vi "CRYPIC Change Sate.vi"(11 "sAction":string) -> (3 "sData_Out":string)   [LabVIEW 2013]
uses:
  CRYMain Sub Window Global.vi
  DataView/VIEW/CRYNew View Global.vi
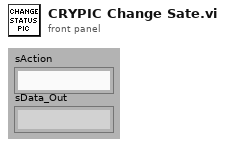
[diagram p1: front panel]
types:
  T1 = enum8{"Enabled", "Disabled", "Disabled and Grayed Out"}
  T2 = typedef "Graph Main Info Cluster.ctl" = cluster{"Selected_BarIdx":i32, "Selected_PanelIdx":i32, "Graph Main VIRef":refnum<vi>, "ToolBarClick":bool, "Spliter Ref Array":refnum<vi>[], "Panel Ref Array":refnum<vi>[], "Spliter_matrix":i32[][], "Panel_matrix":i32[][], "child_spliterIdx_matrix":i32[][], "split_pos_matrix":i32[][], "Title State":bool, "sQueueName":string, "Frame nID":i32, "Graph VIRef Array":cluster{"Graph VIRef":refnum<vi>, "Panel Idx":i32, "Frame VIRef":refnum<vi>, "Icon Ring":i32, "Graph Type":string}[], "View Type":string}
  T3 = typedef "LVRectTypeDef.ctl" = cluster{"Left":i16, "Top":i16, "Right":i16, "Bottom":i16}
  T4 = cluster{"nID":i32[], "Frame":cluster{"nType":i32, "nParent":i32, "pVIW":refnum<vi>, "pSPW":refnum<vi>, "nTypeF":i32, "pVIF":refnum<vi>, "pSPF":refnum<vi>, "nIDSpliter":i32, "nProperty":i32, "Bound":T3, "nID":i32, "nData":i32, "sData":string, "pWVI":refnum<vi>, "sTitle":string, "cPages":cluster{"nPage":i32, "sTitle":string, "sIcon":string, "pVI":refnum<vi>, "nID":i32}[], "pTab":refnum<vi>, "nIDPages":i32[], "pSPT":refnum<vi>, "sTemp":string, "nDockID":i32, "nDockLR":i32, "sIcon":string}[]}
  T5 = cluster{"nType":i32, "nParent":i32, "pVIW":refnum<vi>, "pSPW":refnum<vi>, "nTypeF":i32, "pVIF":refnum<vi>, "pSPF":refnum<vi>, "nIDSpliter":i32, "nProperty":i32, "Bound":T3, "nID":i32, "nData":i32, "sData":string, "pWVI":refnum<vi>, "sTitle":string, "cPages":cluster{"nPage":i32, "sTitle":string, "sIcon":string, "pVI":refnum<vi>, "nID":i32}[], "pTab":refnum<vi>, "nIDPages":i32[], "pSPT":refnum<vi>, "sTemp":string, "nDockID":i32, "nDockLR":i32, "sIcon":string}[]
  T6 = cluster{"Graph VIRef":refnum<vi>, "Panel Idx":i32, "Frame VIRef":refnum<vi>, "Icon Ring":i32, "Graph Type":string}[]
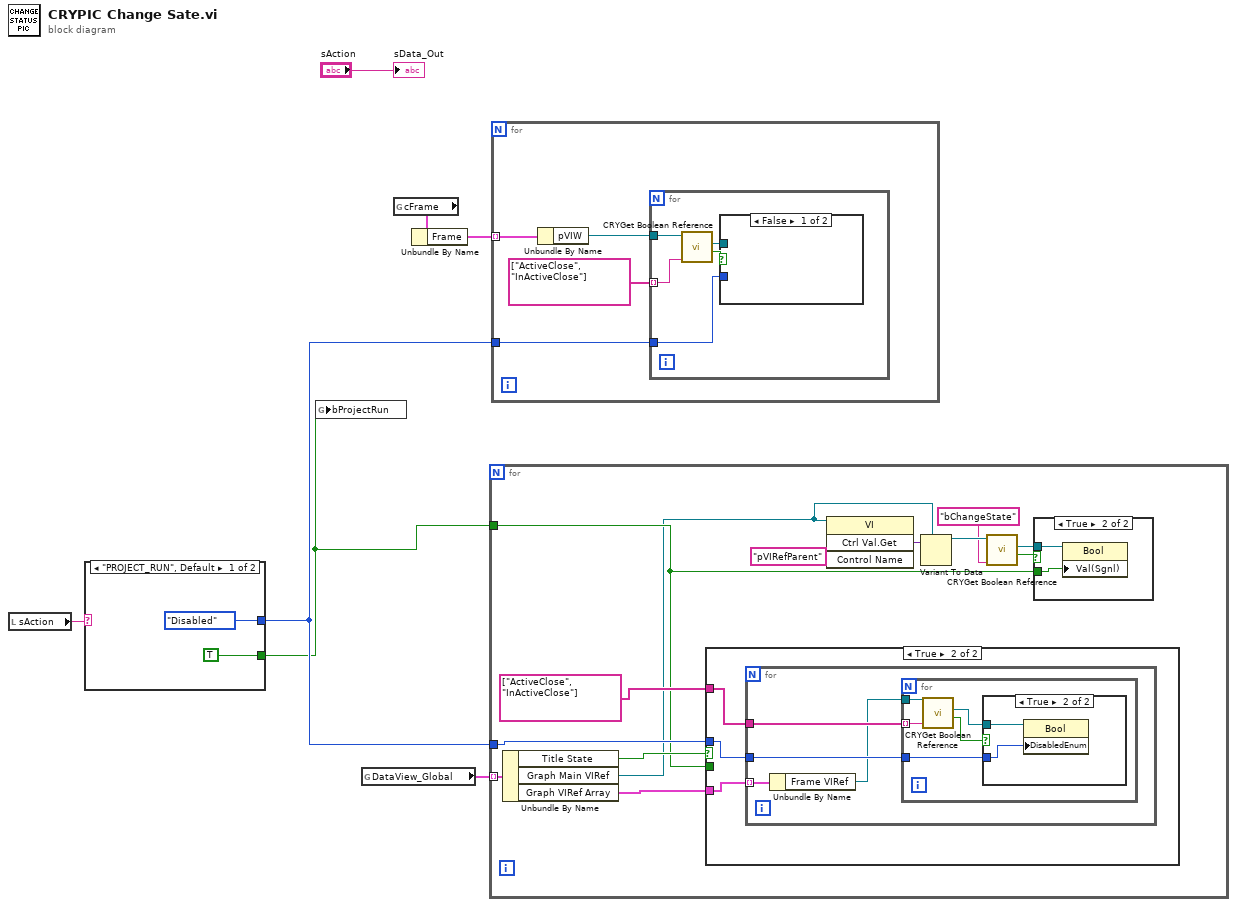
[diagram p0: block diagram]
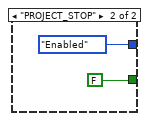
[diagram p5: hidden frame]
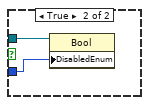
[diagram p6: hidden frame]
diagram:
  n1 = local read "sAction"() -> (w5:string)
  n2 = case shown="\"PROJECT_RUN\", Default" w5 {
    tunnel: [T1."Disabled" ("Disabled") T1."Enabled" ("Disabled")] -> w4
    tunnel: [TRUE ("bProjectRun") FALSE ("bProjectRun")] -> w3
    frame "PROJECT_RUN", Default {
    }
    frame "PROJECT_STOP" {
    }
  }
  n3 = global write "CRYMain Sub Window Global.vi" "bProjectRun"(w3) -> ()
  n4 = global read "CRYNew View Global.vi" "DataView_Global"() -> (w1:T2[])
  n5 = global read "CRYMain Sub Window Global.vi" "cFrame"() -> (w7:T4)
  n6 = Unbundle By Name(w7) -> ("Frame"=w6:T5)
  n7 = for {
    tunnel: w4 -> [w21]
    tunnel: w3 -> [w13]
    tunnel: w1 -> [w24] mode=indexing
    n8 = Unbundle By Name(w24) -> ("Title State"=w23:bool, "Graph Main VIRef"=w12:refnum<vi>, "Graph VIRef Array"=w20:T6)
    n9 = case shown="True" w23 {
      tunnel: string[] ["ActiveClose", "InActiveClose"] -> [_ w29]
      tunnel: w21 -> [_ w28]
      tunnel: w13 -> [_ _]
      tunnel: w20 -> [_ w27]
      frame False {
      }
      frame True {
        n10 = for {
          tunnel: w29 -> [w33]
          tunnel: w28 -> [w32]
          tunnel: w27 -> [w31] mode=indexing
          n11 = Unbundle By Name(w31) -> ("Frame VIRef"=w30:refnum<vi>)
          n12 = for {
            tunnel: w33 -> [w38] mode=indexing
            tunnel: w32 -> [w37]
            tunnel: w30 -> [w36]
            n13 = call "CRYGet Boolean Reference.vi"("Label Name"=w38, "VI Refnum"=w36) -> ("Exist?"=w35:bool, "Boolean Ref"=w34:refnum<vi>)  [unwired: 7 in, 1 out]
            n14 = case shown="True" w35 {
              tunnel: w34 -> [_ w40]
              tunnel: w37 -> [_ w39]
              frame False {
              }
              frame True {
                n15 = property class="Bool"(reference=w40, "DisabledEnum"=w39) -> ()  [unwired: 1 in, 2 out]
              }
            }
          }
        }
      }
    }
    n16 = invoke class="VI" method="Ctrl Val.Get"(reference=w12, "Control Name"="pVIRefParent") -> ("Get Control Value Variant"=w15:variant)  [unwired: 2 in, 3 out]
    n17 = Variant To Data(type=w12, Variant=w15) -> (data=w19:refnum<vi>)  [unwired: 1 in, 1 out]
    n18 = call "CRYGet Boolean Reference.vi"("Label Name"="bChangeState", "VI Refnum"=w19) -> ("Exist?"=w17:bool, "Boolean Ref"=w16:refnum<vi>)  [unwired: 7 in, 1 out]
    n19 = case shown="True" w17 {
      tunnel: w16 -> [_ w26]
      tunnel: w13 -> [_ w25]
      frame False {
      }
      frame True {
        n20 = property class="Bool"(reference=w26, "Val(Sgnl)"=w25) -> ()  [unwired: 1 in, 2 out]
      }
    }
  }
  n21 = for {
    tunnel: w6 -> [w44] mode=indexing
    tunnel: w4 -> [w41]
    n22 = Unbundle By Name(w44) -> ("pVIW"=w43:refnum<vi>)
    n23 = for {
      tunnel: w43 -> [w49]
      tunnel: string[] ["ActiveClose", "InActiveClose"] -> [w48] mode=indexing
      tunnel: w41 -> [w45]
      n24 = call "CRYGet Boolean Reference.vi"("Label Name"=w48, "VI Refnum"=w49) -> ("Exist?"=w47:bool, "Boolean Ref"=w46:refnum<vi>)  [unwired: 7 in, 1 out]
      n25 = case shown="False" w47 {
        tunnel: w46 -> [_ w51]
        tunnel: w45 -> [_ w50]
        frame False {
        }
        frame True {
          n26 = property class="Bool"(reference=w51, "DisabledEnum"=w50) -> ()  [unwired: 1 in, 2 out]
        }
      }
    }
  }
  "sData_Out" <- "sAction"
